vi "SECoP_dataGetAdditionalString.vi"(7 "Position":u32, 8 "error in (no error)":errorcluster, 9 "Index":u32, 10 "SECoP_dataPtr":T1 {"ptr64" format="%.0x"; "ptr32" format="%.0x"}, 11 "DLL path (in)":T2) -> (0 "error out":errorcluster, 2 "Value":string, 3 "DLL path (out)":T2)   [LabVIEW 2023, in "SECoP.lvlib"]
doc: "Call <b>\"SECoP_dataGetAdditionalString.vi\"</b> to retrieve the string value of an additional item of SECoP_dataPtr, selected by index.\n\n<b>DLL path</b> input and output of cluster from \"SECoP-Initialize.vi\"\n<b>SECoP_dataPtr</b> data to access\n<b>Position</b> points to a virtual flattened entry of the data type\n<b>Index</b> zero based index to additional item of SECoP_dataPtr\n<b>Value</b> numeric value"
uses:
  SECoP.lvlib
  SECoP-libraries.ctl
  SECoP-data.ctl
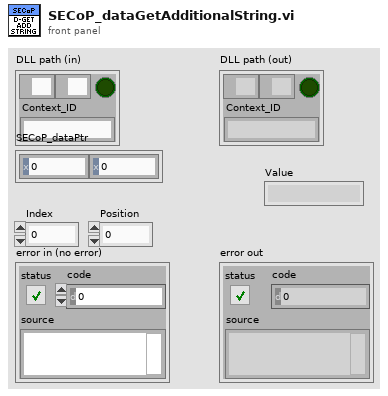
[diagram p1: front panel]
types:
  T1 = typedef "SECoP.lvlib/SECoP-data.ctl" = cluster{"ptr32":u32, "ptr64":u64}
  T2 = typedef "SECoP.lvlib/SECoP-libraries.ctl" = cluster{"serverDLL":path, "variantDLL":path, "cleanup_mode":bool, "Context_ID":string}
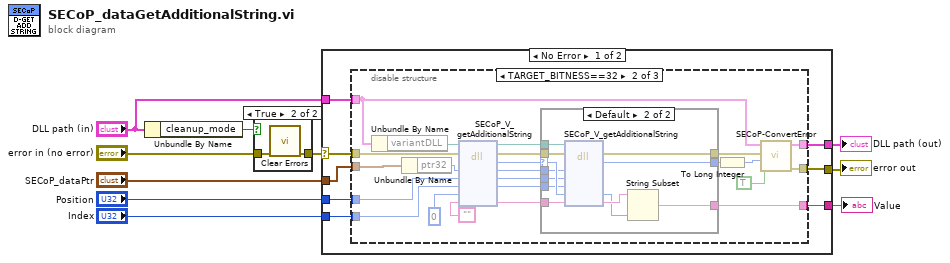
[diagram p0: block diagram]
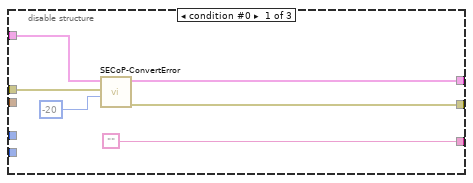
[diagram p3: hidden frame]
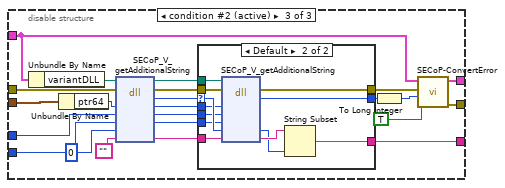
[diagram p5: hidden frame]
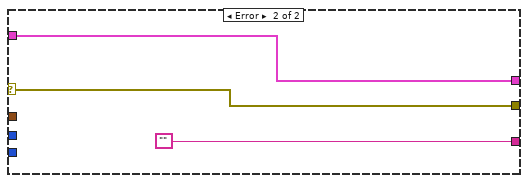
[diagram p7: hidden frame]
diagram:
  n1 = Unbundle By Name("DLL path (in)") -> ("cleanup_mode"=w8:bool)
  n2 = case shown="True" w8 {
    tunnel: "error in (no error)" -> [w11 w13]
    tunnel: [w11 w12] -> w6
    frame False {
    }
    frame True {
      n3 = call <vilib>:"Clear Errors.vi"("error in (no error)"=w13) -> ("error out"=w12:errorcluster)  [unwired: 5 in, 1 out]
    }
  }
  n4 = case shown="No Error" w6 {
    selector: w6 -> [w21 w105]
    tunnel: "DLL path (in)" -> [w15 w106]
    tunnel: [w17 w106] -> w10
    tunnel: [w18 w105] -> w9
    tunnel: "Position" -> [w20 _]
    tunnel: [w19 ""] -> w4
    tunnel: "SECoP_dataPtr" -> [w16 _]
    tunnel: "Index" -> [w14 _]
    frame No Error {
      n5 = disable-structure shown="TARGET_BITNESS==32" {
        disable-tunnel: w21 -> [w24 w50 w88]
        disable-tunnel: w20 -> [_ w49 w87]
        disable-tunnel: ["" w40 w78] -> w19
        disable-tunnel: [w26 w34 w72] -> w18
        disable-tunnel: [w27 w35 w73] -> w17
        disable-tunnel: w16 -> [_ w47 w85]
        disable-tunnel: w15 -> [w25 w29 w66]
        disable-tunnel: w14 -> [_ w31 w69]
        frame condition #0 {
          n6 = call "SECoP-ConvertError.vi"("return code"=-20, "error in (no error)"=w24, "DLL path (in)"=w25) -> ("error out"=w26:errorcluster, "DLL path (out)"=w27:T2)  [unwired: 7 in]
        }
        frame condition #1 {
          n7 = Unbundle By Name(w29) -> ("variantDLL"=w28:path)
          n8 = Unbundle By Name(w47) -> ("ptr32"=w46:u32)
          n9 = dll-call lib="Z:/Praktische_Aufgaben/SECoP-LabVIEW2015/32bit/SECoP32.dll" fn="SECoP_V_getAdditionalString"(path in=w28, error in=w50, "pData"=w46, "uPosition"=w49, "uIndex"=w31, "uBufferSize"=u32 0 ("BufferSize"), "pValue"="") -> (path out=w43:path, error out=w42:errorcluster, "return type"=w44:u32, "pData"=w33:u32, "uPosition"=w32:u32, "uIndex"=w30:u32, "pValue"=w41:string)  [unwired: 2 in]
          n10 = case shown="Default" w44 {
            selector: w44 -> [w52 w62]
            tunnel: w43 -> [_ w65]
            tunnel: w42 -> [w53 w64]
            tunnel: [w53 w63] -> w36
            tunnel: [w52 w61] -> w37
            tunnel: w41 -> [w51 w60]
            tunnel: [w51 w57] -> w40
            tunnel: w33 -> [_ w56]
            tunnel: w32 -> [_ w55]
            tunnel: w30 -> [_ w54]
            frame 0 {
            }
            frame Default {
              n11 = dll-call lib="Z:/Praktische_Aufgaben/SECoP-LabVIEW2015/32bit/SECoP32.dll" fn="SECoP_V_getAdditionalString"(path in=w65, error in=w64, "pData"=w56, "uPosition"=w55, "uIndex"=w54, "uBufferSize"=w62, "pValue"=w60) -> (error out=w63:errorcluster, "return type"=w61:u32, "uBufferSize"=w58:u32, "pValue"=w59:string)  [unwired: 4 in, 1 out]
              n12 = String Subset(string=w59, length (rest)=w58) -> (substring=w57:string)  [unwired: 1 in]
            }
          }
          n13 = To Long Integer(number=w37) -> (32bit integer=w38:i32)
          n14 = call "SECoP-ConvertError.vi"("return is boolean"=TRUE, "return code"=w38, "error in (no error)"=w36, "DLL path (in)"=w29) -> ("error out"=w34:errorcluster, "DLL path (out)"=w35:T2)  [unwired: 6 in]
        }
        frame condition #2 (active) {
          n15 = Unbundle By Name(w66) -> ("variantDLL"=w67:path)
          n16 = Unbundle By Name(w85) -> ("ptr64"=w84:u64)
          n17 = dll-call lib="Z:/Praktische_Aufgaben/SECoP-LabVIEW2015/32bit/SECoP32.dll" fn="SECoP_V_getAdditionalString"(path in=w67, error in=w88, "pData"=w84, "uPosition"=w87, "uIndex"=w69, "uBufferSize"=u32 0 ("BufferSize"), "pValue"="") -> (path out=w81:path, error out=w80:errorcluster, "return type"=w82:u32, "pData"=w71:u64, "uPosition"=w70:u32, "uIndex"=w68:u32, "pValue"=w79:string)  [unwired: 2 in]
          n18 = case shown="Default" w82 {
            selector: w82 -> [w90 w100]
            tunnel: w81 -> [_ w103]
            tunnel: w80 -> [w91 w102]
            tunnel: [w91 w101] -> w74
            tunnel: [w90 w99] -> w75
            tunnel: w79 -> [w89 w98]
            tunnel: [w89 w95] -> w78
            tunnel: w71 -> [_ w94]
            tunnel: w70 -> [_ w93]
            tunnel: w68 -> [_ w92]
            frame 0 {
            }
            frame Default {
              n19 = dll-call lib="Z:/Praktische_Aufgaben/SECoP-LabVIEW2015/32bit/SECoP32.dll" fn="SECoP_V_getAdditionalString"(path in=w103, error in=w102, "pData"=w94, "uPosition"=w93, "uIndex"=w92, "uBufferSize"=w100, "pValue"=w98) -> (error out=w101:errorcluster, "return type"=w99:u32, "uBufferSize"=w96:u32, "pValue"=w97:string)  [unwired: 4 in, 1 out]
              n20 = String Subset(string=w97, length (rest)=w96) -> (substring=w95:string)  [unwired: 1 in]
            }
          }
          n21 = To Long Integer(number=w75) -> (32bit integer=w76:i32)
          n22 = call "SECoP-ConvertError.vi"("return is boolean"=TRUE, "return code"=w76, "error in (no error)"=w74, "DLL path (in)"=w66) -> ("error out"=w72:errorcluster, "DLL path (out)"=w73:T2)  [unwired: 6 in]
        }
      }
    }
    frame Error {
    }
  }
  "DLL path (out)" <- w10
  "error out" <- w9
  "Value" <- w4
